vi "Analyseur de spectre.vi"() -> ()   [LabVIEW 2013]
uses:
  <vilib>/measure/NI_MAPro.lvlib
  <instrlib>/niUSRP/niUSRP Fetch Rx Data (CDB WDT).vi
  <vilib>/measure/maspectr.llb/FFT Power Spectrum and PSD for 1 Chan (CDB).vi
  <vilib>/measure/maspectr.llb/Power Spectrum and PSD Export Mode.ctl
panel:
  in  "export mode":T1 caption="mode d'exportation" items=["Spectre de puissance", "Densité spectrale de puissance"]
  in  "averaging parameters":T2={"averaging mode"=enum."No averaging", "weighting mode"=enum."Exponential", "number of averages"=10} caption="paramètres de moyennage" {"number of averages" min=1}
  in  "Stop Button":bool
  out "Frequency Plot":cluster{"f0":dbl, "df":dbl, "magnitude":dbl[]}(graph)
  in  "device names":refnum<k15>="192.168.10.3"
  in  "active antenna":string="RX1"
  in  "timeout":dbl=10.0
  in  "number of samples":i64=10000
  out "error out":errorcluster
  out "coerced gain":dbl=10.0 format="%#_6f"
  out "coerced carrier frequency":dbl=315000000.0 format="%#_6p"
  out "coerced IQ rate":dbl=5000000.0 format="%#_6p"
  in  "gain":dbl=10.0 format="%#_6f"
  in  "carrier frequency":dbl=915000000.0 format="%#_6p"
  in  "IQ rate":dbl=1000000.0 format="%#_6p"
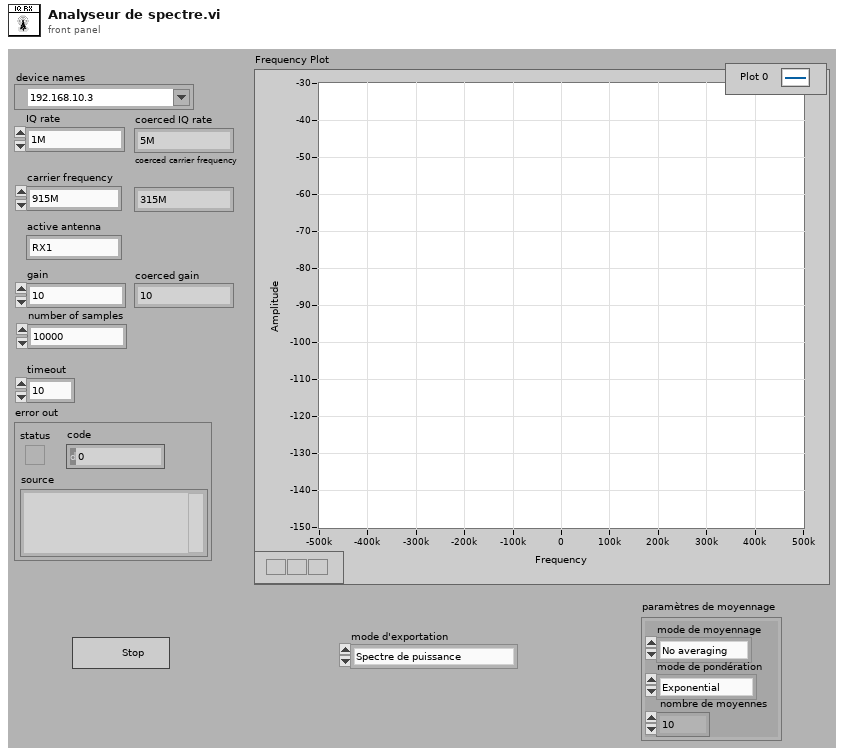
[diagram p1: front panel]
types:
  T1 = typedef "NI_MAPro.lvlib/Power Spectrum and PSD Export Mode.ctl" = u16
  T2 = cluster{"averaging mode":enum16{"No averaging", "Vector averaging", "RMS averaging", "Peak hold"}, "weighting mode":enum16{"Linear", "Exponential"}, "number of averages":u32}
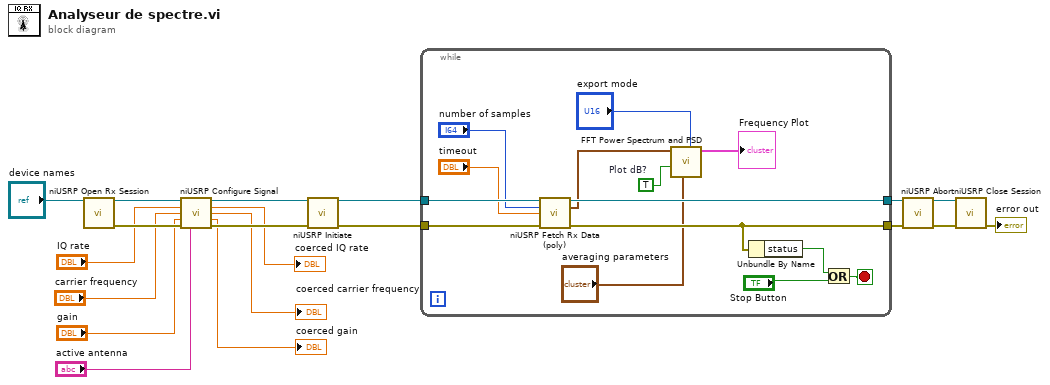
[diagram p0: block diagram]
diagram:
  n1 = call <instrlib>:"niUSRP Open Rx Session.vi"("device names"="device names") -> ("session handle out"=w18:refnum<k15>, "error out"=w17:errorcluster)  [unwired: 13 in]
  n2 = call <instrlib>:"niUSRP Configure Signal.vi"("session handle"=w18, "IQ rate"="IQ rate", "carrier frequency"="carrier frequency", "gain"="gain", "error in (no error)"=w17, "active antenna"="active antenna") -> ("session handle out"=w7:refnum<k15>, "coerced IQ rate"=→"coerced IQ rate":dbl, "coerced carrier frequency"=→"coerced carrier frequency":dbl, "coerced gain"=→"coerced gain":dbl, "error out"=w9:errorcluster)  [unwired: 5 in]
  n3 = call <instrlib>:"niUSRP Initiate.vi"("session handle"=w7, "error in (no error)"=w9) -> ("session handle out"=w13:refnum<k15>, "error out"=w12:errorcluster)  [unwired: 12 in]
  n4 = while {
    tunnel: w13 -> [w33]
    tunnel: w12 -> [w32]
    tunnel: [w27] -> w2
    tunnel: [w26] -> w1
    stop <- w25 stop-if-true
    w28 = TRUE  # Plot dB?
    n5 = call-poly <instrlib>:"niUSRP Fetch Rx Data (poly).vi"("session handle"=w33, "number of samples"="number of samples", "timeout"="timeout", "error in (no error)"=w32) -> ("session handle out"=w27:refnum<k15>, "data"=w22:waveform(cdb), "error out"=w26:errorcluster)  [unwired: 8 in, 1 out]
    n6 = call-poly <vilib>:"FFT Power Spectrum and PSD.vi"("export mode"="export mode", "averaging parameters"="averaging parameters", "dB On (F)"=w28, "time signal"=w22) -> ("Power Spectrum / PSD"=→"Frequency Plot":cluster{"f0":dbl, "df":dbl, "magnitude":dbl[]})  [unwired: 4 in, 3 out]
    n7 = Unbundle By Name(w26) -> ("status"=w31:bool)
    n8 = Or(x=w31, y="Stop Button") -> (x .or. y?=w25:bool)
  }
  n9 = call <instrlib>:"niUSRP Abort.vi"("session handle"=w2, "error in (no error)"=w1) -> ("session handle out"=w15:refnum<k15>, "error out"=w14:errorcluster)  [unwired: 12 in]
  n10 = call <instrlib>:"niUSRP Close Session.vi"("session handle"=w15, "error in (no error)"=w14) -> ("error out"=→"error out":errorcluster)  [unwired: 13 in]
